vi "Labspec PutDataInfo.vi"(6 "Table Entry":u16(ring) items=["Integration time", "Number of accumulations", "Frequency", "Hole size", "Slit size", "Laser", "Grating", "Filter", "Spectral Width", "Detector", "Detector Size", "Operator", "Sample", "Remark", "Power"], 7 "Table Name":u16(ring) items=["Acquisition", "Custom"], 8 "error in":errorcluster, 9 "TableValue":string, 10 "DataID":i32, 11 "Automation Refnum In":refnum<k7>) -> (0 "error out":errorcluster, 3 "Automation Refnum Out":refnum<k7>)   [LabVIEW 2014]
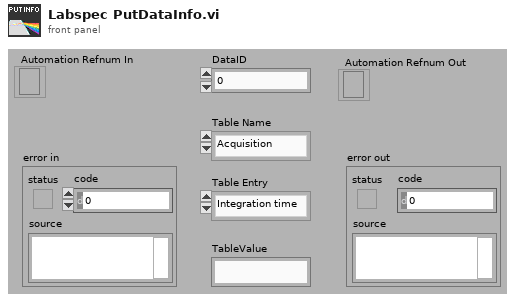
[diagram p1: front panel]
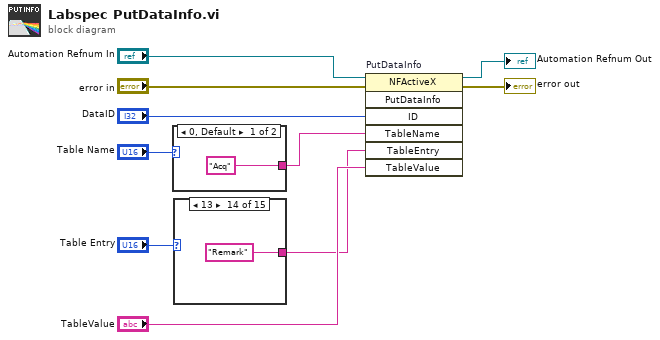
[diagram p0: block diagram]
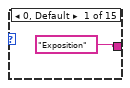
[diagram p2: hidden frame]
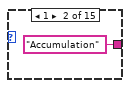
[diagram p3: hidden frame]
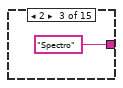
[diagram p4: hidden frame]
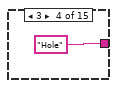
[diagram p5: hidden frame]
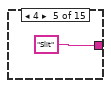
[diagram p6: hidden frame]
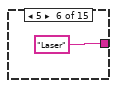
[diagram p7: hidden frame]
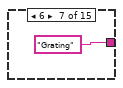
[diagram p8: hidden frame]
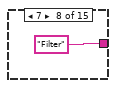
[diagram p9: hidden frame]
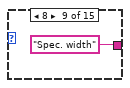
[diagram p10: hidden frame]
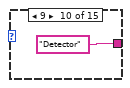
[diagram p11: hidden frame]
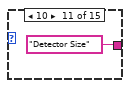
[diagram p12: hidden frame]
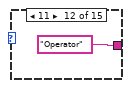
[diagram p13: hidden frame]
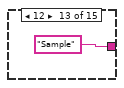
[diagram p14: hidden frame]
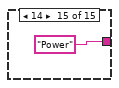
[diagram p15: hidden frame]
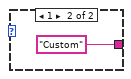
[diagram p16: hidden frame]
diagram:
  n1 = case shown="0, Default" "Table Name" {
    tunnel: ["Acq" "Custom"] -> w4
    frame 0, Default {
    }
    frame 1 {
    }
  }
  n2 = case shown="13" "Table Entry" {
    tunnel: ["Exposition" "Accumulation" "Spectro" "Hole" "Slit" "Laser" "Grating" "Filter" "Spec. width" "Detector" "Detector Size" "Operator" "Sample" "Remark" "Power"] -> w1
    frame 0, Default {
    }
    frame 1 {
    }
    frame 2 {
    }
    frame 3 {
    }
    frame 4 {
    }
    frame 5 {
    }
    frame 6 {
    }
    frame 7 {
    }
    frame 8 {
    }
    frame 9 {
    }
    frame 10 {
    }
    frame 11 {
    }
    frame 12 {
    }
    frame 13 {
    }
    frame 14 {
    }
  }
  n3 = invoke on="PutDataInfo" class="NFActiveX" method="PutDataInfo"(reference="Automation Refnum In", error in="error in", "ID"="DataID", "TableName"=w4, "TableEntry"=w1, "TableValue"="TableValue") -> (reference out=→"Automation Refnum Out":refnum<k7>, error out=→"error out":errorcluster)  [unwired: 1 in, 5 out]
